vi "SubVI_LiftyBoi_Teleop.vi"(8 "error in (no error)":errorcluster, 9 "Buttons":bool[](array[boolean]), 10 "Axes":dbl[](array[numeric]), 11 "TeleOp Elapsed Seconds":dbl) -> (0 "error out":errorcluster)   [LabVIEW 2017]
uses:
  <vilib>/Rock Robotics/WPI/ThirdParty/Phoenix-LabVIEW/Motor Controller/Controls/CTRE_Phoenix_MotorControl_ControlMode.ctl
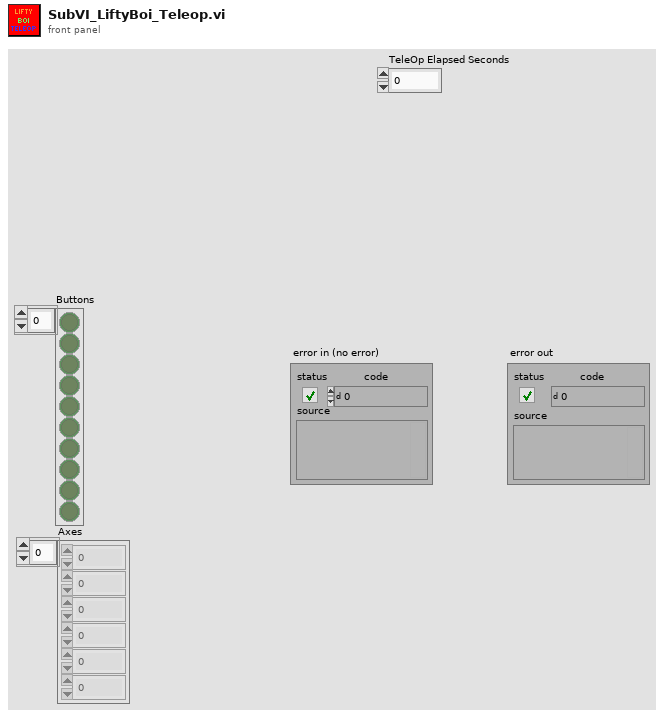
[diagram p1: front panel]
types:
  T1 = typedef "CTRE_Phoenix_MotorControl_ControlMode.ctl" = u16
  T2 = typedef "WPI_MotorControlDeviceRef.ctl" = cluster{"DeviceStatus":errorcluster, "Type":T3, "PWM":cluster{"PWM Channel":T4, "DeadBand":T5}, "CAN":cluster{"Device Number":u8, "SetOutput VI Ref":variant, "GetOutput VI Ref":variant, "Enable VI Ref":variant, "Disable VI Ref":variant, "Data":variant}, "Invert":bool, "DIO PWM":cluster{"PWM \"Enable\" Channel":T4, "DIOChannel":T6, "PWM Rate":dbl}}
  T3 = typedef "WPI_MotorControlType.ctl" = enum16{"PWM", "CAN", "DIO PWM"}
  T4 = typedef "FPGA_DIOPWMChannel.ctl" = enum8{"PWM 0", "PWM 1", "PWM 2", "PWM 3", "PWM 4", "PWM 5", "PWM 6", "PWM 7", "PWM 8", "PWM 9", "PWM MXP 0", "PWM MXP 1", "PWM MXP 2", "PWM MXP 3", "PWM MXP 4", "PWM MXP 5", "PWM MXP 6", "PWM MXP 7", "PWM MXP 8", "PWM MXP 9", "Invalid"}
  T5 = typedef "WPI_PWMDeadband.ctl" = cluster{"Name":string, "maxPositivePwm":i32, "minPositivePwm":i32, "centerPwm":i32, "maxNegativePwm":i32, "minNegativePwm":i32, "angularRange":u16}
  T6 = typedef "FPGA_DIOChannel.ctl" = enum8{"DIO 0", "DIO 1", "DIO 2", "DIO 3", "DIO 4", "DIO 5", "DIO 6", "DIO 7", "DIO 8", "DIO 9", "DIO MXP 0", "DIO MXP 1", "DIO MXP 2", "DIO MXP 3", "DIO MXP 4", "DIO MXP 5", "DIO MXP 6", "DIO MXP 7", "DIO MXP 8", "DIO MXP 9", "DIO MXP 10", "DIO MXP 11", "DIO MXP 12", "DIO MXP 13", "DIO MXP 14", "DIO MXP 15", "SPI Port CS1", "SPI Port CS2", "SPI Port CS3", "SPI Port MISO", "SPI Port MOSI", "Invalid"}
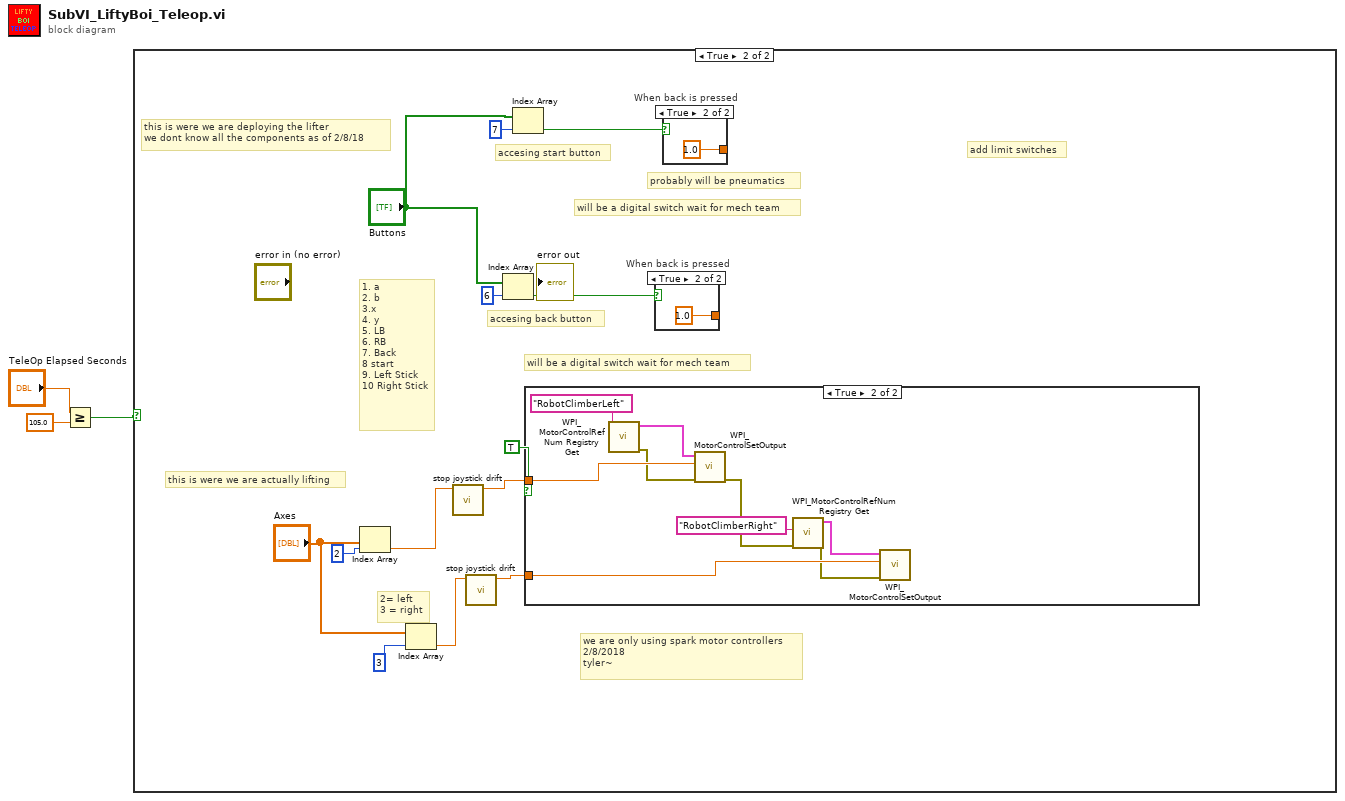
[diagram p0: block diagram]
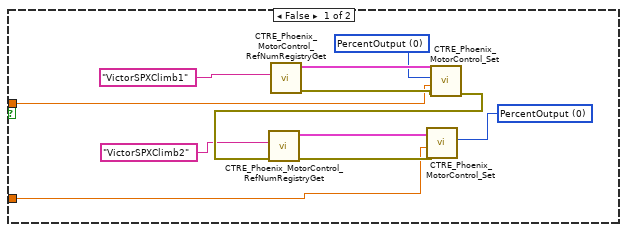
[diagram p3: hidden frame]
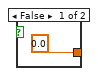
[diagram p4: hidden frame]
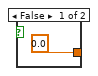
[diagram p5: hidden frame]
diagram:
  n1 = Greater Or Equal?(x="TeleOp Elapsed Seconds", y=105.0) -> (x >= y?=w1:bool)
  n2 = case shown="True" w1 {
    frame False {
    }
    frame True {
      # "this is were we are actually lifting"
      # "add limit switches"
      # "this is were we are deploying the lifter\nwe dont know all the components as of 2/8/18"
      # "we are only using spark motor controllers\n2/8/2018\ntyler~"
      # "2= left\n3 = right"
      # "probably will be pneumatics"
      # "will be a digital switch wait for mech team"
      # "accesing start button"
      # "will be a digital switch wait for mech team"
      # "accesing back button"
      # "1. a\n2. b\n3.x \n4. y\n5. LB \n6. RB\n7. Back\n8 start\n9. Left Stick\n10 Right Stick"
      n3 = Index Array(array="Axes", index=2) -> (element=w10:dbl)
      n4 = Index Array(array="Axes", index=3) -> (element=w5:dbl)
      n5 = call "stop joystick drift.vi"("upper limit in"=w10) -> ("upper limit out"=w9:dbl)  [unwired: 10 in]
      n6 = call "stop joystick drift.vi"("upper limit in"=w5) -> ("upper limit out"=w8:dbl)  [unwired: 10 in]
      n7 = Index Array(array="Buttons", index=6) -> (element=w15:bool)
      n8 = Index Array(array="Buttons", index=7) -> (element=w12:bool)
      n9 = case shown="True" TRUE ("Boolean") {
        tunnel: w9 -> [w20 w36]
        tunnel: w8 -> [w19 w33]
        frame False {
          w17 = T1 0 items=["PercentOutput"=0, "Position"=1, "Velocity"=2, "Current"=3, "Follower"=5, "MotionProfile"=6, "MotionMagic"=7, "MotionMagicArc"=8, "MotionProfileArc"=10, "Disabled"=15] ("Control Mode")
          w18 = T1 0 items=["PercentOutput"=0, "Position"=1, "Velocity"=2, "Current"=3, "Follower"=5, "MotionProfile"=6, "MotionMagic"=7, "MotionMagicArc"=8, "MotionProfileArc"=10, "Disabled"=15] ("Control Mode")
          n10 = call <vilib>:"CTRE_Phoenix_MotorControl_RefNumRegistryGet.vi"("refnum name"="VictorSPXClimb1") -> ("error out"=w25:errorcluster, "PhoenixMotorControlDevRef"=w27:T2)  [unwired: 9 in]
          n11 = call <vilib>:"CTRE_Phoenix_MotorControl_Set.vi"("error in (no error)"=w25, "Output"=w20, "Control Mode"=w17, "PhoenixMotorControlDevRef"=w27) -> ("error out"=w23:errorcluster)  [unwired: 6 in, 1 out]
          n12 = call <vilib>:"CTRE_Phoenix_MotorControl_RefNumRegistryGet.vi"("error in (no error)"=w23, "refnum name"="VictorSPXClimb2") -> ("error out"=w24:errorcluster, "PhoenixMotorControlDevRef"=w26:T2)  [unwired: 8 in]
          n13 = call <vilib>:"CTRE_Phoenix_MotorControl_Set.vi"("error in (no error)"=w24, "Output"=w19, "Control Mode"=w18, "PhoenixMotorControlDevRef"=w26) -> ()  [unwired: 6 in, 2 out]
        }
        frame True {
          n14 = call <vilib>:"WPI_MotorControlRefNum Registry Get.vi"("refnum name"="RobotClimberLeft") -> ("error out"=w29:errorcluster, "MotorControlDevRef"=w35:T2)  [unwired: 9 in]
          n15 = call <vilib>:"WPI_MotorControlSetOutput.vi"("error in (no error)"=w29, "Output"=w36, "MotorControlDevRef"=w35) -> ("error out"=w28:errorcluster)  [unwired: 6 in, 2 out]
          n16 = call <vilib>:"WPI_MotorControlRefNum Registry Get.vi"("error in (no error)"=w28, "refnum name"="RobotClimberRight") -> ("error out"=w30:errorcluster, "MotorControlDevRef"=w32:T2)  [unwired: 8 in]
          n17 = call <vilib>:"WPI_MotorControlSetOutput.vi"("error in (no error)"=w30, "Output"=w33, "MotorControlDevRef"=w32) -> ()  [unwired: 6 in, 3 out]
        }
      }
      n18 = case "When back is pressed" shown="True" w15 {
        tunnel: [0.0 1.0 ("Output")] -> _
        frame False {
        }
        frame True {
        }
      }
      n19 = case "When back is pressed" shown="True" w12 {
        tunnel: [0.0 1.0 ("Output")] -> _
        frame False {
        }
        frame True {
        }
      }
    }
  }
